vi "TALOS Config Param.vi"(6 "Load":bool, 8 "error in (no error)":errorcluster, 11 "Parameter Name":string) -> (0 "error out":errorcluster, 3 "Output":string)   [LabVIEW 2026, in "TALOS.lvlib"]
doc: "This VI stores in memory all the configuration parameters of TALOS loaded at startup from TALOS_Config_Param.ini ."
uses:
  TALOS.lvlib
  Ancestor/Ancestor/Ancestor.lvclass/Ancestor.ctl
  FGV/Error Memory/Get Error Description.vi
  Get PC name.vi
  Ancestor/Ancestor/Read ID.vi
  Get Class Name.vi
  <vilib>/Utility/error.llb/Clear Errors.vi
  FGV/Error Memory/Error Memory Core.vi
  <vilib>/AdvancedString/Delimited String to 1D String Array.vi
  <vilib>/AdvancedString/Delimited String to 1D String Array (string).vi
  Circus Root Path.vi
  FGV/Error Memory/Error Crt Lvl checker.vi
  FGV/Error Memory/Error Memory Core.vi/40c8088d-b597-4017-91af-faa98e00292e.vi
  FGV/Error Memory/Error Memory Core.vi/d4a3ab98-063c-4e44-b43d-fbdcfe6c2be2.vi
  Global Memory.vi
  <vilib>/Utility/LVClass/Get LV Class Name.vi
  Is in Packed Library.vi
  Read CSV worksheet.vi
  Global Constants.vi
  <vilib>/Utility/error.llb/General Error Handler.vi
  <vilib>/Utility/config.llb/Read Key (String).vi
  Ancestor/Ancestor/Ancestor.lvclass
  <vilib>/Comparison/Equal/Equal Functor/Equal Functor.lvclass
  <vilib>/Utility/config.llb/NI_LVConfig.lvlib
panel:
  out "key names":string[][](array[string])
  out "section names":string[](array[string])
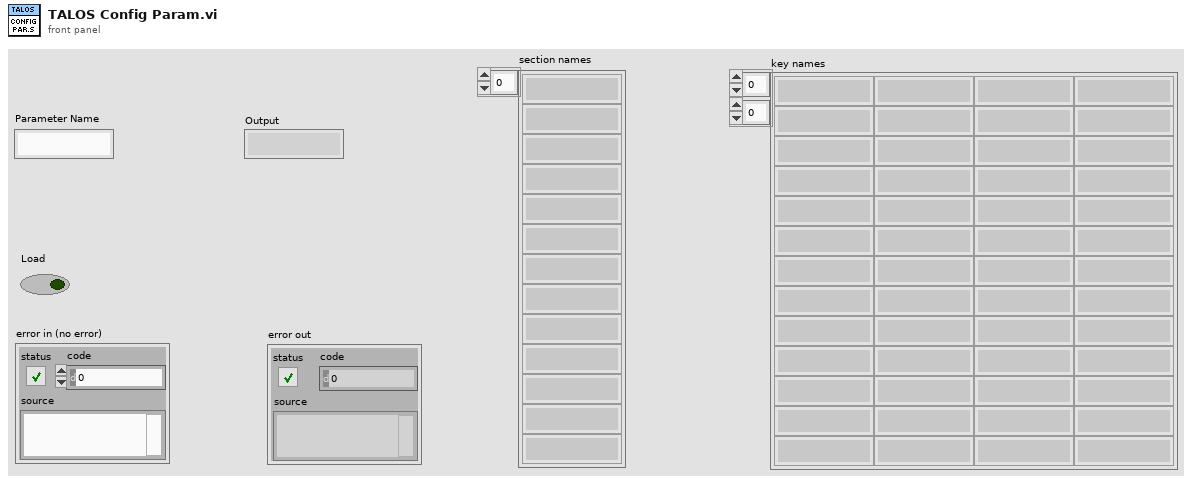
[diagram p1: front panel]
types:
  T1 = typedef "NI_LVConfig.lvlib/Config Data RefNum.ctl" = refnum<k1>
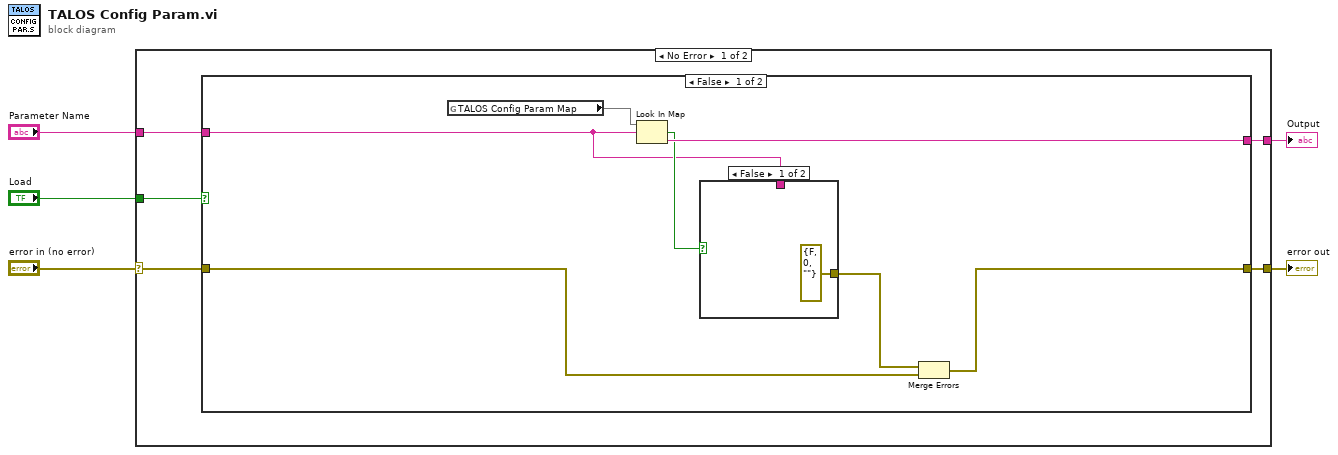
[diagram p0: block diagram]
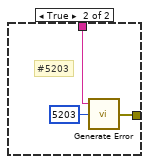
[diagram p2: hidden frame]
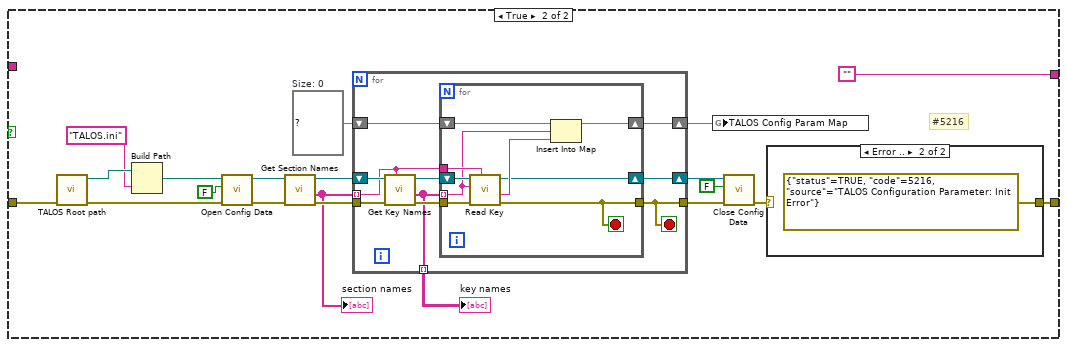
[diagram p3: hidden frame]
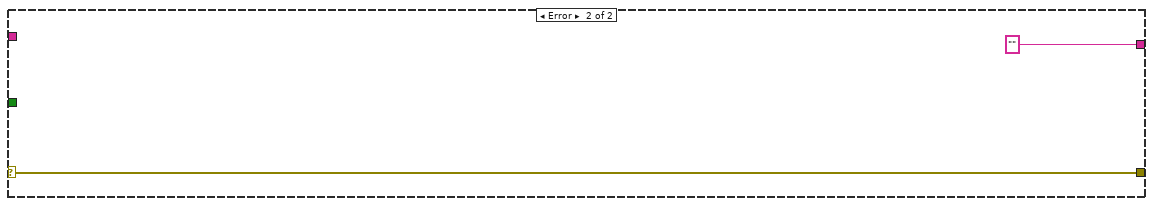
[diagram p5: hidden frame]
diagram:
  n1 = case shown="No Error" "error in (no error)" {
    selector: "error in (no error)" -> [w9 w64]
    tunnel: "Load" -> [w10 _]
    tunnel: [w8 w64] -> w3
    tunnel: [w7 "" ("Output")] -> w2
    tunnel: "Parameter Name" -> [w6 _]
    frame No Error {
      n2 = case shown="False" w10 {
        tunnel: w9 -> [w17 w26]
        tunnel: [w15 w23] -> w8
        tunnel: [w16 "" ("Output")] -> w7
        tunnel: w6 -> [w11 _]
        frame False {
          n3 = global read "Global Memory.vi" "TALOS Config Param Map"() -> (w12:map{string, string})
          n4 = Look In Map(map=w12, key=w11) -> (key not found?=w14:bool, value=w16:string)  [unwired: 1 in]
          n5 = case shown="False" w14 {
            tunnel: [errorcluster {"status"=FALSE, "code"=0, "source"=""} ("error constant") w20] -> w13
            tunnel: w11 -> [_ w19]
            frame False {
            }
            frame True {
              # "#5203"
              n6 = call "Generate Error.vi"("Optional String"=w19, "Error Code"=5203) -> ("error out"=w20:errorcluster)  [unwired: 5 in]
            }
          }
          n7 = Merge Errors(w13, w17) -> (w15:errorcluster)
        }
        frame True {
          w25 = map{string, string} {}  # Size: 0
          # "#5216"
          n8 = call "TALOS Root path.vi"("error in (no error)"=w26) -> ("error out"=w27:errorcluster, "TALOS Root Path"=w30:path)  [unwired: 9 in]
          n9 = Build Path(base path=w30, name or relative path="TALOS.ini") -> (appended path=w28:path)
          n10 = call <vilib>:"Open Config Data.vi"("error in (no error)"=w27, "create file if necessary (T)"=FALSE, "configuration file path"=w28) -> ("error out"=w40:errorcluster, "refnum"=w39:T1)  [unwired: 6 in, 1 out]
          n11 = call <vilib>:"Get Section Names.vi"("error in (no error)"=w40, "refnum"=w39) -> ("error out"=w37:errorcluster, "section names"=w36:string[], "refnum out"=w38:T1)  [unwired: 7 in]
          "section names" <- w36
          n12 = for {
            tunnel: w37 -> [w52]
            tunnel: w36 -> [w49] mode=indexing
            tunnel: [w48] -> w35 mode=indexing
            tunnel: [w44] -> w34
            shift-right: [w47] -> w22
            shift-left: w25 -> [w46]
            shift-right: [w45] -> w33
            shift-left: w38 -> [w53]
            stop <- w44 stop-if-true
            n13 = call <vilib>:"Get Key Names.vi"("section"=w49, "error in (no error)"=w52, "refnum"=w53) -> ("error out"=w50:errorcluster, "key names"=w48:string[], "refnum out"=w51:T1)  [unwired: 5 in, 1 out]
            n14 = for {
              tunnel: w50 -> [w61]
              tunnel: w49 -> [w60]
              tunnel: w48 -> [w59] mode=indexing
              tunnel: [w54] -> w44
              shift-right: [w57] -> w47
              shift-left: w46 -> [w56]
              shift-right: [w55] -> w45
              shift-left: w51 -> [w62]
              stop <- w54 stop-if-true
              n15 = call-poly <vilib>:"Read Key.vi"("section"=w60, "error in (no error)"=w61, "key"=w59, "refnum"=w62) -> ("error out"=w54:errorcluster, "value"=w58:string, "refnum out"=w55:T1)  [unwired: 4 in, 1 out]
              n16 = Insert Into Map(map in=w56, key=w59, value=w58) -> (map out=w57:map{string, string})  [unwired: 2 out]
            }
          }
          "key names" <- w35
          n17 = global write "Global Memory.vi" "TALOS Config Param Map"(w22) -> ()
          n18 = call <vilib>:"Close Config Data.vi"("error in (no error)"=w34, "write file if changed (T)"=FALSE, "refnum"=w33) -> ("error out"=w24:errorcluster)  [unwired: 7 in, 1 out]
          n19 = case shown="Error .." w24 {
            selector: w24 -> [w42 _]
            tunnel: [w42 errorcluster {"status"=TRUE, "code"=5216, "source"="TALOS Configuration Parameter: Init Error"} ("error IO")] -> w23
            frame No Error {
            }
            frame Error {
            }
          }
        }
      }
    }
    frame Error {
    }
  }
  "error out" <- w3
  "Output" <- w2
